vi "Controller Load Configuration.vi"(8 "error in (no error)":errorcluster, 11 "FOFB Configuration Path":path) -> (0 "error out":errorcluster, 3 "FOFB Configuration":T1={"FOFB Parameters"={"Network"={"FOFB Controller IP"="", "LNLS Control Network IP"="", "LNLS Control Network Power Supplies TCP Port"=0, "LNLS Control Network FOFB Configuration TCP Port"=0, "LNLS Control Network BPMs TCP Port"=0, "Monitoring Data TCP Port"=0, "Fast Archiver TCP Port"=0, "Fast Command TCP Port"=0, "TCP Listening Timeout"=0}, "Fast Acquisition"={"Sampling Period"=0, "Data Buffer Size"=0, "Monitoring Period"=0}, "Acquisition Network"=[], "Actuation Network"=[]}, "Number of Acquisition Chassis"=0, "Number of Actuation Chassis"=0, "Number of BPM Readings"=0, "BPM Reading Names"=[], "Selected BPM Readings"=[0, 1, 2, 3, 4, 5, 6, 7, 8, 9, 10, 11, 12, 13, 14, 15, 16, 17, 18, 19, 20, 21, 22, 23, 24, 25, 26, 27, 28, 29, 30, 31, 32, 33, 34, 35, 36, 37, 38, 39, 40, 41, 42, 43, 44, 45, 46, 47, 48, 49], "Number of Correctors"=0, "Corrector Names"=[], "Selected Correctors"=[0, 1, 2, 3, 4, 5, 6, 7, 8, 9, 10, 11, 12, 13, 14, 15, 16, 17, 18, 19, 20, 21, 22, 23, 24, 25, 26, 27, 28, 29, 30, 31, 32, 33, 34, 35, 36, 37, 38, 39, 40, 41, 42, 43, 44, 45, 46, 47, 48, 49], "Response Matrix"=[], "Reference Orbit"=[], "Correction Matrix"=[], "FPGA Filter Sets"=[], "Acquisition Chassis Names"=[], "Actuation Chassis Names"=[], "Acquisition Variables"=[], "Actuation Variables"=[], "PS Matrix Mapping"=[], "Inverse PS Matrix Mapping"=[], "BPM Matrix Mapping"=[], "Inverse BPM Matrix Mapping"=[], "BPM Planes"=[], "Corrector Planes"=[]})   [LabVIEW 2011, in "Controller VIs.lvlib"]
doc: "Load the FOFB Controller configuration and parameters from a configuration file and builds the configuration cluster (FOFB Configuration) used thorough the program execution. Perform tasks related with the FOFB configuration, such as change of Scan Engine period, load response matrix from file, load reference orbit from file, calculate correction matrix."
uses:
  Controller VIs.lvlib
  Types Definitions/Type FOFB Configuration.ctl
  Types Definitions/Type FOFB Parameters.ctl
  Types Definitions/Type Network Configuration.ctl
  Types Definitions/Type FA Configuration.ctl
  Types Definitions/Type Acquisition Network Configuration.ctl
  Types Definitions/Type Actuation Network Configuration.ctl
  XML VIs.lvlib
  Type Definitions.lvlib
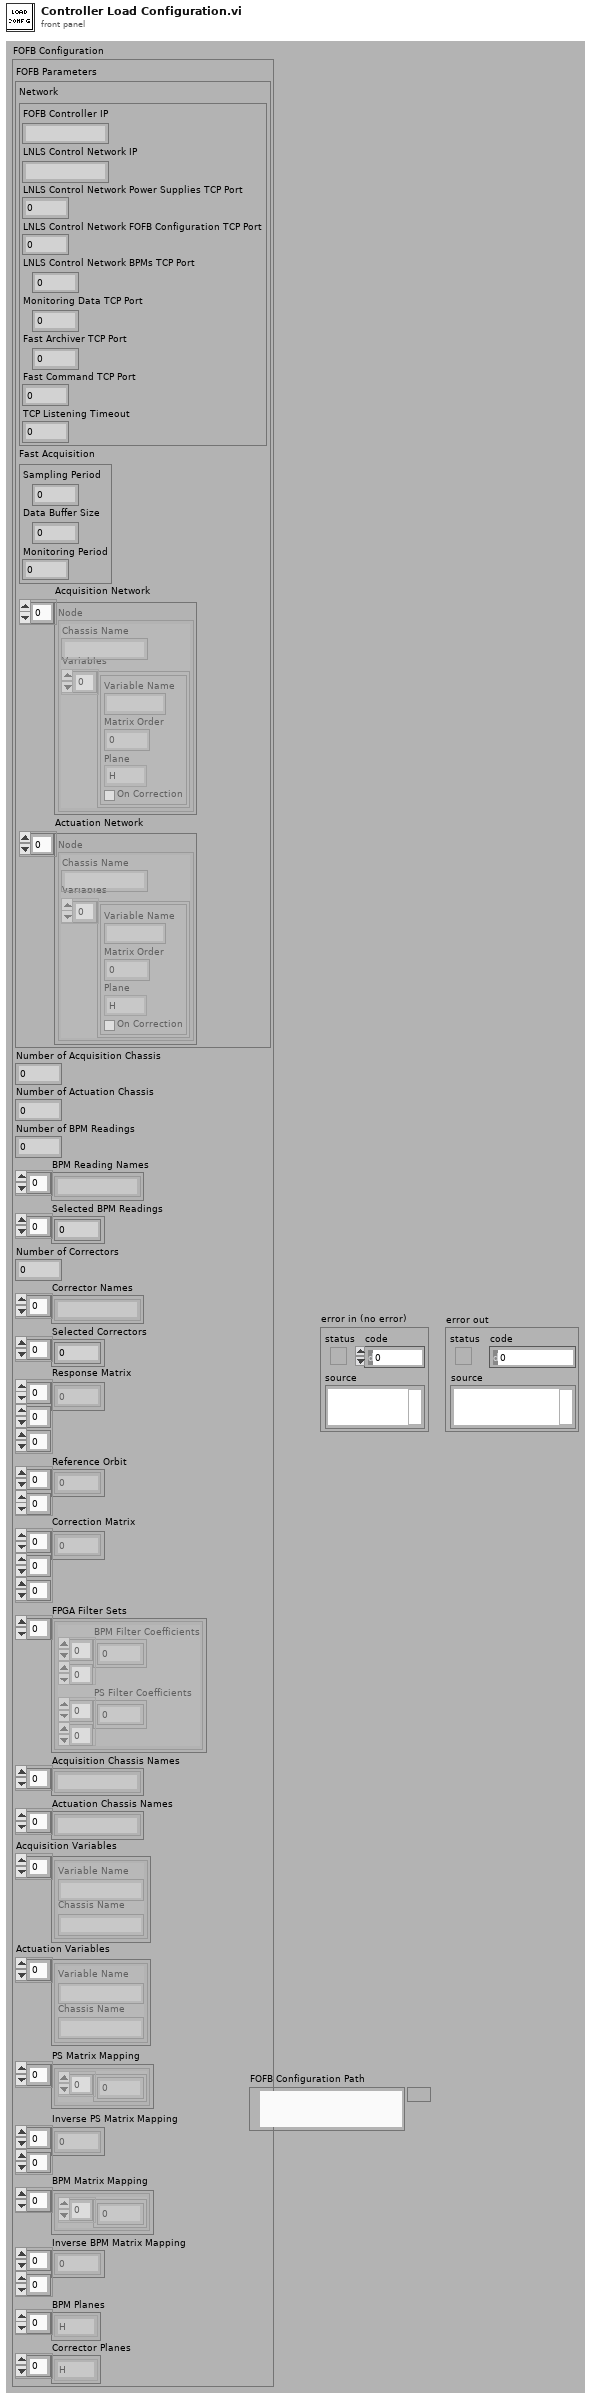
[diagram p1: front panel]
types:
  T1 = typedef "Type Definitions.lvlib/Type FOFB Configuration.ctl" = cluster{"FOFB Parameters":T2, "Number of Acquisition Chassis":i32, "Number of Actuation Chassis":i32, "Number of BPM Readings":i32, "BPM Reading Names":string[], "Selected BPM Readings":u32[], "Number of Correctors":i32, "Corrector Names":string[], "Selected Correctors":u32[], "Response Matrix":dbl[][][], "Reference Orbit":dbl[][], "Correction Matrix":dbl[][][], "FPGA Filter Sets":cluster{"BPM Filter Coefficients":dbl[][], "PS Filter Coefficients":dbl[][]}[], "Acquisition Chassis Names":string[], "Actuation Chassis Names":string[], "Acquisition Variables":cluster{"Variable Name":string, "Chassis Name":string}[], "Actuation Variables":cluster{"Variable Name":string, "Chassis Name":string}[], "PS Matrix Mapping":cluster{u32[]}[], "Inverse PS Matrix Mapping":u32[][], "BPM Matrix Mapping":cluster{u32[]}[], "Inverse BPM Matrix Mapping":u32[][], "BPM Planes":enum8{"H", "V"}[], "Corrector Planes":enum8{"H", "V"}[]}
  T2 = typedef "Type Definitions.lvlib/Type FOFB Parameters.ctl" = cluster{"Network":T3, "Fast Acquisition":T4, "Acquisition Network":T5, "Actuation Network":T6}
  T3 = typedef "Type Definitions.lvlib/Type Network Configuration.ctl" = cluster{"FOFB Controller IP":string, "LNLS Control Network IP":string, "LNLS Control Network Power Supplies TCP Port":u16, "LNLS Control Network FOFB Configuration TCP Port":u16, "LNLS Control Network BPMs TCP Port":u16, "Monitoring Data TCP Port":u16, "Fast Archiver TCP Port":u16, "Fast Command TCP Port":u16, "TCP Listening Timeout":i32}
  T4 = typedef "Type Definitions.lvlib/Type FA Configuration.ctl" = cluster{"Sampling Period":u32, "Data Buffer Size":u32, "Monitoring Period":u32}
  T5 = typedef "Type Definitions.lvlib/Type Acquisition Network Configuration.ctl" = cluster{"Chassis Name":string, "Variables":cluster{"Variable Name":string, "Matrix Order":u32, "Plane":enum8{"H", "V"}, "On Correction":bool}[]}[]
  T6 = typedef "Type Definitions.lvlib/Type Actuation Network Configuration.ctl" = cluster{"Chassis Name":string, "Variables":cluster{"Variable Name":string, "Matrix Order":u32, "Plane":enum8{"H", "V"}, "On Correction":bool}[]}[]
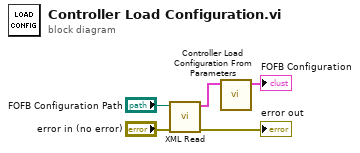
[diagram p0: block diagram]
diagram:
  n1 = call "XML Read.vi"("error in"="error in (no error)", "XML File Path In"="FOFB Configuration Path") -> ("error out"=→"error out":errorcluster, "FOFB Parameters"=w4:T2)  [unwired: 8 in]
  n2 = call "Controller Load Configuration From Parameters.vi"("FOFB Parameters"=w4) -> ("FOFB Configuration"=→"FOFB Configuration":T1)  [unwired: 9 in, 1 out]
